vi "Create.vi"(9 "Start Position":cluster{"Row":i32, "Col":i32}, 10 "Input":string) -> (3 "Proto":refnum<class "Proto.lvclass">)   [LabVIEW 2021, in "Proto.lvclass"]
uses:
  Proto.lvclass
  Direction.ctl
  Proto.lvclass/Proto.ctl
  Helpers/Helpers.lvlib
panel:
  out "Array":i32[][](array[numeric])
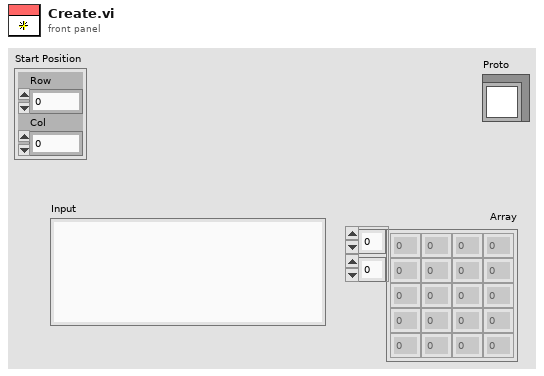
[diagram p1: front panel]
types:
  T1 = typedef "Proto.lvclass/Direction.ctl" = enum16{"Up", "Down", "Right", "Left"}
  T2 = map{cluster{"Row":i32, "Col":i32}, set{cluster{"Heat":i32, "Prev Steps":T1[]}}}
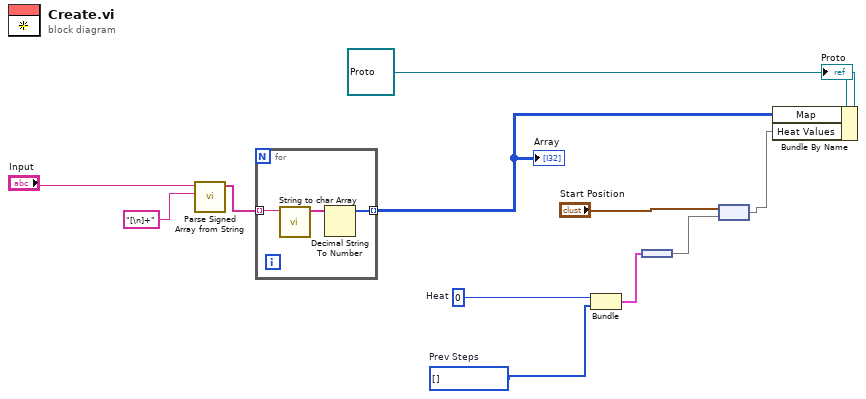
[diagram p0: block diagram]
diagram:
  w5 = 0  # Heat
  w4 = T1[] [] items=["Up", "Down", "Right", "Left"]  # Prev Steps
  n1 = call "Parse Signed Array from String.vi"("Delimiter regex"="[\n]+", "Input"="Input") -> ("Parsed Array"=w9:string[])  [unwired: 8 in, 1 out]
  n2 = for {
    tunnel: w9 -> [w15] mode=indexing
    tunnel: [w13] -> w7 mode=indexing
    n3 = call "String to char Array.vi"("Row"=w15) -> ("Array"=w14:string[])  [unwired: 10 in]
    n4 = Decimal String To Number(string=w14) -> (number=w13:i32[])  [unwired: 2 in, 1 out]
  }
  "Array" <- w7
  n5 = Bundle("Heat"=w5, "Prev Steps"=w4) -> (w3:cluster{"Heat":i32, "Prev Steps":T1[]})  [unwired: 1 in]
  n6 = node(w3) -> (w2:set{cluster{"Heat":i32, "Prev Steps":T1[]}})
  n7 = node("Start Position", w2) -> (w1:T2)
  n8 = Bundle By Name(cluster=refnum<class "Proto.lvclass"> refnum ("Proto"), "Map"=w7, "Heat Values"=w1) -> (→"Proto":refnum<class "Proto.lvclass">)
